vi "DynamicIOCMDCore.vi"(9 "New_Write_CMD":T1={"Data"=0.0, "Register"="", "DataType"="", "Address"="", "Protocol"="", "IOAddress"={"Register"=0, "Address"=0, "Device"=0, "Length"=0, "Offset"=0}, "WriteMode"="0"}, 10 "DeviceIndex":i32, 11 "Function":enum16{"INIT", "NEW", "GET"}(ring)) -> (1 "NewCMD":T1[](array[typedef]), 3 "Have new write CMD":bool)   [LabVIEW 2020, in "DynamicIOCMD.lvlib"]
uses:
  DynamicIOCMD.lvlib
  DynamicIOCMD.ctl
panel:
  out "Buffer":cluster{"Device":T1[]}[](array[cluster])
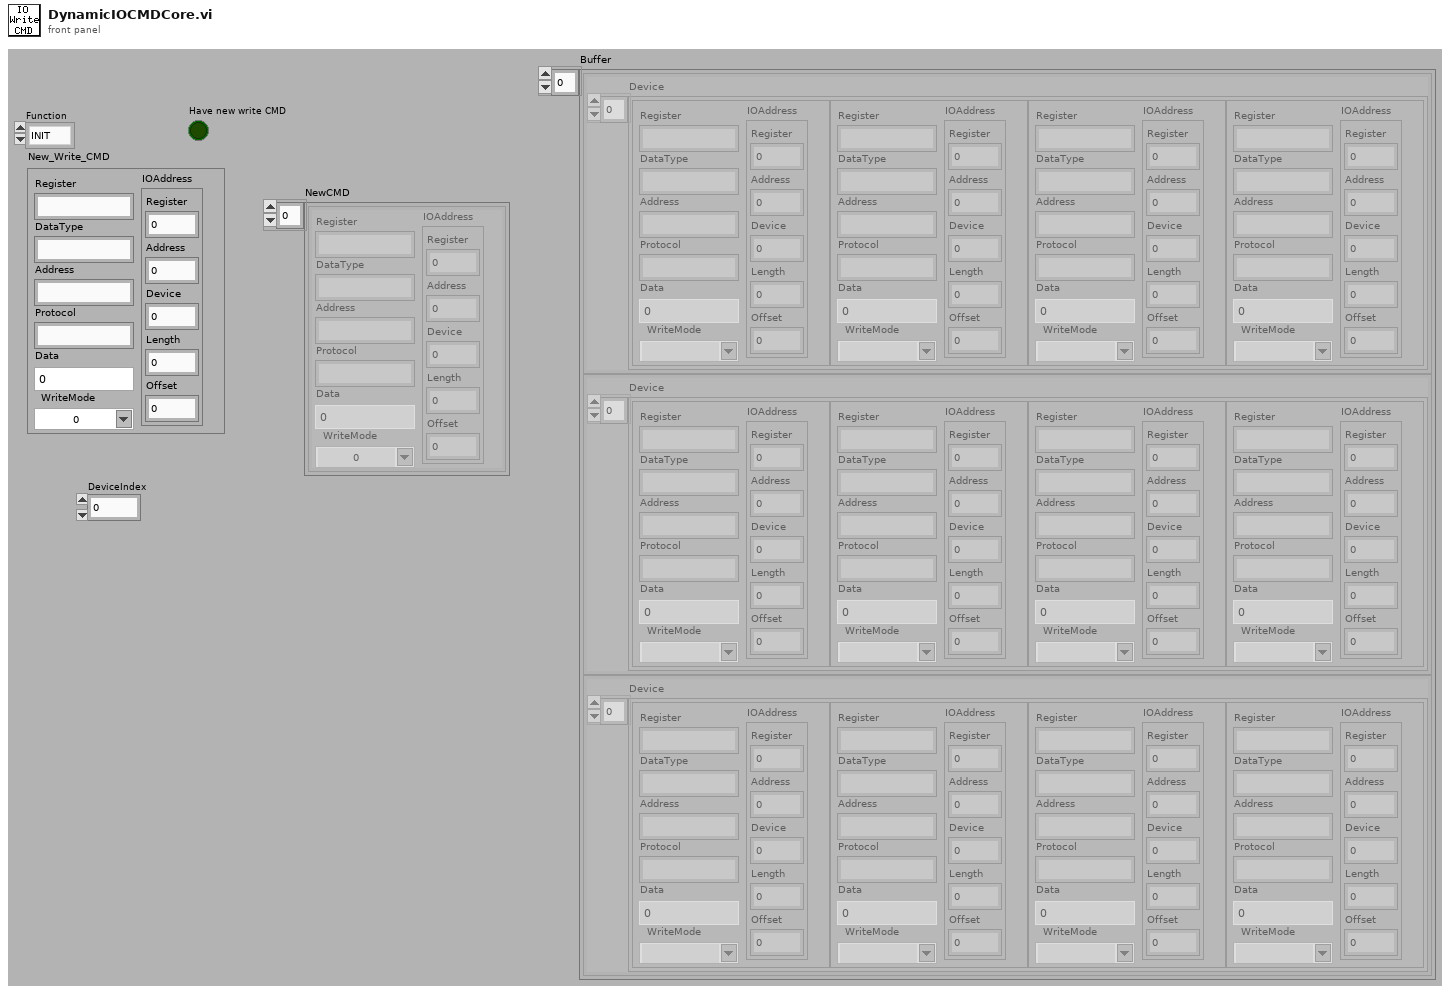
[diagram p1: front panel]
types:
  T1 = typedef "DynamicIOCMD.lvlib/DynamicIOCMD.ctl" = cluster{"Data":dbl, "Register":string, "DataType":string, "Address":string, "Protocol":string, "IOAddress":cluster{"Register":i32, "Address":i32, "Device":i32, "Length":i32, "Offset":i32}, "WriteMode":string}
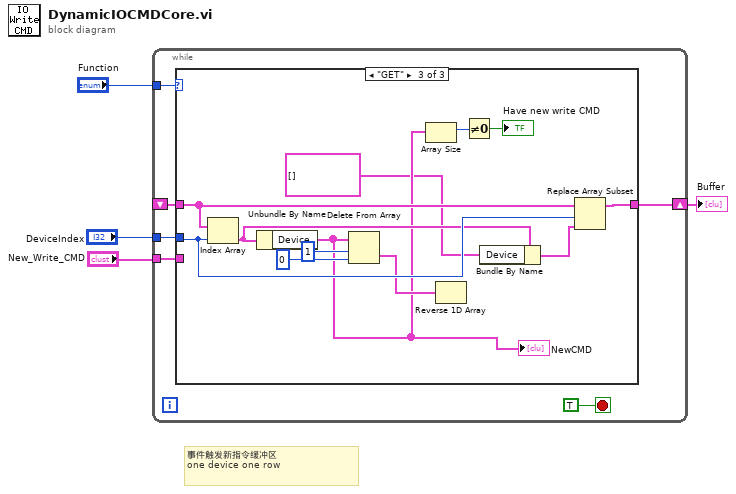
[diagram p0: block diagram]
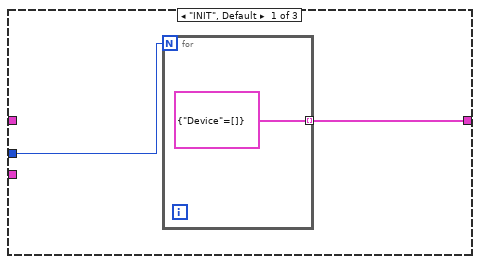
[diagram p2: hidden frame]
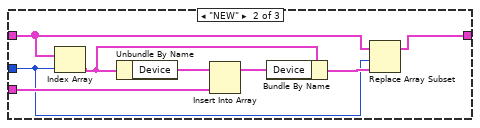
[diagram p3: hidden frame]
diagram:
  # "事件触发新指令缓冲区\none device one row"
  n1 = while {
    tunnel: "Function" -> [w9]
    shift-right: [w8] -> w1
    shift-left: _ -> [w6]
    tunnel: "New_Write_CMD" -> [w7]
    tunnel: "DeviceIndex" -> [w5]
    stop <- TRUE stop-if-true
    n2 = case shown="\"GET\"" w9 {
      tunnel: [w12 w14 w30] -> w8
      tunnel: w7 -> [_ w20 _]
      tunnel: w6 -> [_ w17 w31]
      tunnel: w5 -> [w11 w15 w29]
      frame "INIT", Default {
        n3 = for {
          N: w11 -> [_]
          tunnel: [cluster{"Device":T1[]} {"Device"=[]}] -> w12 mode=indexing
        }
      }
      frame "NEW" {
        n4 = Index Array(array=w17, index=w15) -> (element=w19:cluster{"Device":T1[]})
        n5 = Unbundle By Name(w19) -> ("Device"=w21:T1[])
        n6 = Insert Into Array(array=w21, new element=w20) -> (w18:T1[])  [unwired: 1 in]
        n7 = Bundle By Name(cluster=w19, "Device"=w18) -> (w16:cluster{"Device":T1[]})
        n8 = Replace Array Subset(array=w17, new element=w16, index=w15) -> (w14:cluster{"Device":T1[]}[])
      }
      frame "GET" {
        n9 = Index Array(array=w31, index=w29) -> (element=w26:cluster{"Device":T1[]})
        n10 = Unbundle By Name(w26) -> ("Device"=w23:T1[])
        "NewCMD" <- w23
        n11 = Delete From Array(array=w23, length=1, index=0) -> (deleted portion=w24:T1[])  [unwired: 1 out]
        n12 = Array Size(array=w23) -> (size(s)=w33:i32)
        n13 = Reverse 1D Array(array=w24) -> ()  [unwired: 1 out]
        n14 = Not Equal To 0?(x=w33) -> (x != 0?=→"Have new write CMD":bool)
        n15 = Bundle By Name(cluster=w26, "Device"=T1[] []) -> (w25:cluster{"Device":T1[]})
        n16 = Replace Array Subset(array=w31, new element=w25, index=w29) -> (w30:cluster{"Device":T1[]}[])
      }
    }
  }
  "Buffer" <- w1
